vi "Load and Save Example-Rq.vi"(8 "error in (no error)":errorcluster, 11 "Control References":refnum<vi>[](array[refnum])) -> (0 "error out":errorcluster)   [LabVIEW 2018]
uses:
  RWC_Actions.ctl
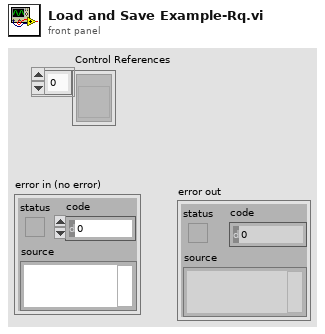
[diagram p1: front panel]
types:
  T1 = typedef "RWC_Actions.ctl" = enum16{"Read", "Write", "Read and Create"}
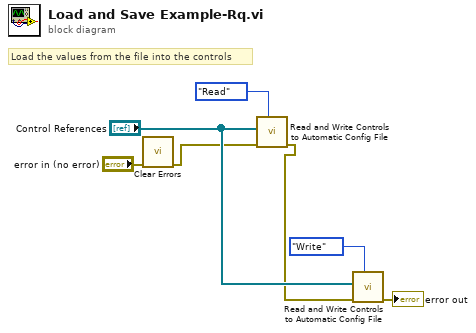
[diagram p0: block diagram]
diagram:
  # "Load the values from the file into the controls"
  n1 = call <vilib>:"Clear Errors.vi"("error in (no error)"="error in (no error)") -> ("error out"=w4:errorcluster)  [unwired: 5 in, 1 out]
  n2 = call "Read and Write Controls to Automatic Config File.vi"("Action"=RWC_Actions."Read", "error in"=w4, "Control References"="Control References") -> ("error out"=w5:errorcluster)  [unwired: 8 in]
  n3 = call "Read and Write Controls to Automatic Config File.vi"("Action"=RWC_Actions."Write", "error in"=w5, "Control References"="Control References") -> ("error out"=→"error out":errorcluster)  [unwired: 8 in]
